vi "Open SystemLink Connection.vi"(5 "SystemLink server base URL":string="https://", 7 "username":string, 9 "password":string, 11 "error in (no error)":errorcluster) -> (4 "SystemLink connection out":T1, 15 "error out":errorcluster)   [LabVIEW 2017, in "SystemLink_States_API.lvlib"]
doc: "Opens an HTTP client handle and passes on the SystemLink server base URL.\n\nInputs:\nSystemLink server base URL- Specifies the base URL of the SystemLink server to connect with (e.g. https://192.168.10.15, https://mysystemlinkserver.com)\nUsername - Specify the SystemLink username\nPassword - Specify the SystemLink password\n\nOutput:\nSystemLink repo out - pass this wire to all the other VIs in this SystemLink Repo API."
uses:
  SystemLink_States_API.lvlib
  _support/systemlink repo.ctl
  <vilib>/httpClient/ClientHandle.ctl
  <vilib>/httpClient/LabVIEWHTTPClient.lvlib
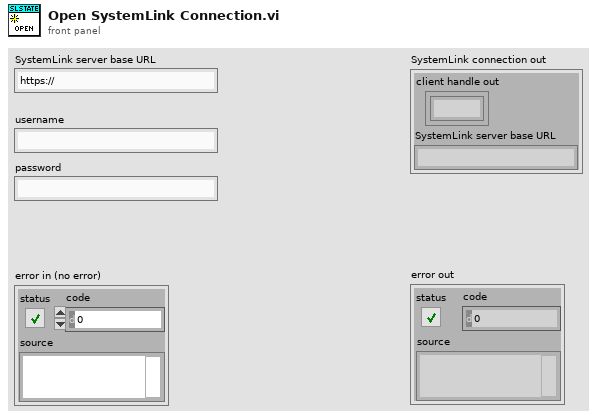
[diagram p1: front panel]
types:
  T1 = typedef "SystemLink_States_API.lvlib/systemlink repo.ctl" = cluster{"client handle out":T2, "SystemLink server base URL":string}
  T2 = typedef "LabVIEWHTTPClient.lvlib/ClientHandle.ctl" = refnum<k1>
  T3 = cluster{"client handle out":T2, "SystemLink server base URL":string}
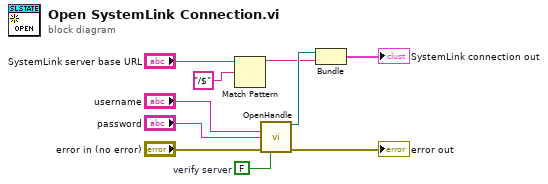
[diagram p0: block diagram]
diagram:
  w8 = FALSE  # verify server
  n1 = Match Pattern(string="SystemLink server base URL", regular expression="/$") -> (before substring=w1:string)  [unwired: 1 in, 3 out]
  n2 = call <vilib>:"OpenHandle.vi"("username"="username", "password"="password", "error in (no error)"="error in (no error)", "verify server(true)"=w8) -> ("client handle out"=w5:T2, "error out"=→"error out":errorcluster)  [unwired: 10 in]
  n3 = Bundle("client handle out"=w5, "SystemLink server base URL"=w1) -> (→"SystemLink connection out":T3)  [unwired: 1 in]
